vi "Find VMR DLL.vi"() -> (2 "error out":errorcluster, 3 "DLL Path":path)   [LabVIEW 2020, in "VoiceMeeterRemote.lvlib" / "VoiceMeeterRemote.lvclass"]
uses:
  VoiceMeeterRemote.lvclass
  <vilib>/Utility/sysdir.llb/System Directory Type.ctl
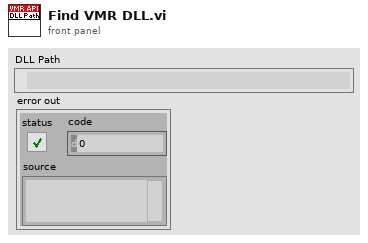
[diagram p1: front panel]
types:
  T1 = typedef "System Directory Type.ctl" = i32
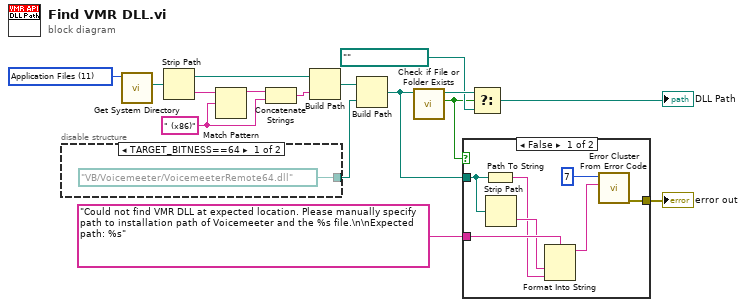
[diagram p0: block diagram]
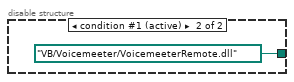
[diagram p3: hidden frame]
diagram:
  w12 = " (x86)" ("regular expression")
  w16 = T1 11 items=["User Home"=0, "User Desktop"=1, "User Documents"=2, "User Application Data"=3, "User Preferences"=4, "User Temporary"=5, "Public Documents"=6, "Public Application Data"=7, "Public Preferences"=8, "Public Cache"=13, "System Core Libraries"=9, "System Installed Libraries"=10, "Application Files"=11, "Boot Volume Root"=12] ("system directory type")
  n1 = disable-structure shown="TARGET_BITNESS==64" {
    disable-tunnel: [path "VB/Voicemeeter/VoicemeeterRemote64.dll" ("name or relative path") path "VB/Voicemeeter/VoicemeeterRemote.dll" ("name or relative path")] -> w4
    frame condition #0 {
    }
    frame condition #1 (active) {
    }
  }
  n2 = call <vilib>:"Get System Directory.vi"("system directory type"=w16) -> ("system directory"=w15:path)  [unwired: 10 in]
  n3 = Strip Path(path=w15) -> (stripped path=w11:path, name=w14:string)
  n4 = Match Pattern(string=w14, regular expression=w12) -> (before substring=w13:string)  [unwired: 1 in, 3 out]
  n5 = Concatenate Strings(w13, w12) -> (w10:string)
  n6 = Build Path(base path=w11, name or relative path=w10) -> (appended path=w9:path)
  n7 = Build Path(base path=w9, name or relative path=w4) -> (appended path=w1:path)
  n8 = call <vilib>:"Check if File or Folder Exists.vi"("path"=w1) -> ("file or folder exists?"=w5:bool, "dup path"=w8:path)  [unwired: 8 in, 1 out]
  n9 = case shown="False" w5 {
    tunnel: w1 -> [w25 _]
    tunnel: "Could not find VMR DLL at expected location. Please manually specify path to installation path of Voicemeeter and the %s file.\n\nExpected path: %s" -> [w24 _]
    tunnel: [w19 _] -> w2
    frame False {
      n10 = Path To String(path=w25) -> (string=w22:string)
      n11 = Strip Path(path=w25) -> (name=w23:string)  [unwired: 1 out]
      n12 = Format Into String(format string=w24, w23, w22) -> (resulting string=w21:string)  [unwired: 2 in, 1 out]
      n13 = call <vilib>:"Error Cluster From Error Code.vi"("error message (\"\")"=w21, "error code (0)"=7) -> ("error out"=w19:errorcluster)  [unwired: 7 in]
    }
    frame True {
    }
  }
  "error out" <- w2
  n14 = Select(t=w8, s=w5, f=path "") -> (s? t:f=→"DLL Path":path)
